vi "PathAtTicket.vi"(0 "Ticket Name":string) -> (8 "path":path)   [LabVIEW 2023]
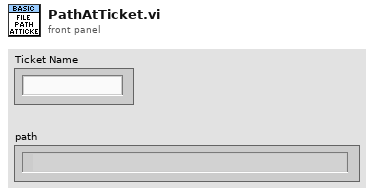
[diagram p1: front panel]
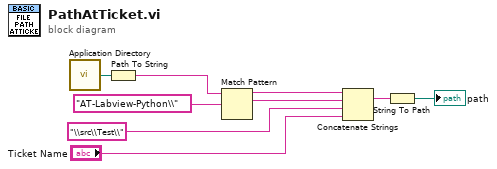
[diagram p0: block diagram]
diagram:
  n1 = call <vilib>:"Application Directory.vi"() -> ("Application Directory"=w9:path)
  n2 = Path To String(path=w9) -> (string=w8:string)
  n3 = Match Pattern(string=w8, regular expression="AT-Labview-Python\\") -> (before substring=w6:string, match substring=w5:string)  [unwired: 1 in, 2 out]
  n4 = Concatenate Strings(w6, w5, "\\src\\Test\\" ("string"), "Ticket Name") -> (w3:string)
  n5 = String To Path(string=w3) -> (path=→"path":path)
